vi "APSxSensorRefCurveLeveling.vi"(8 "error in (no error)":errorcluster caption="错误输入（无错误）", 9 "Param2":dbl, 10 "Param1":enum16{"APSX_PREV_INDEX_POINT_CALIBRATION"}(ring), 11 "hSENSOR":i32) -> (0 "error out":errorcluster caption="错误输出")   [LabVIEW 2018]
doc: "该模板用于创建子VI。"
uses:
  APSx.dll/APSx.dll
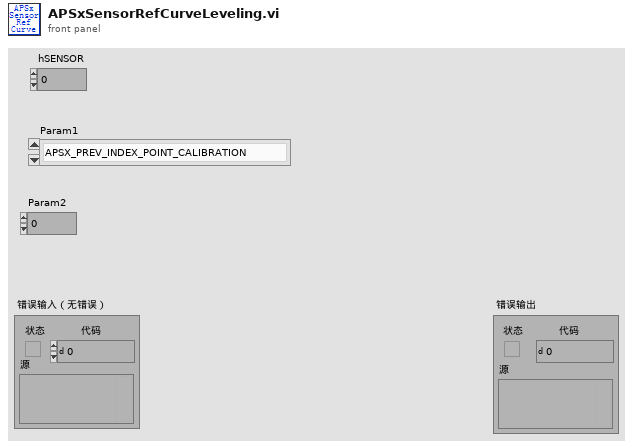
[diagram p1: front panel]
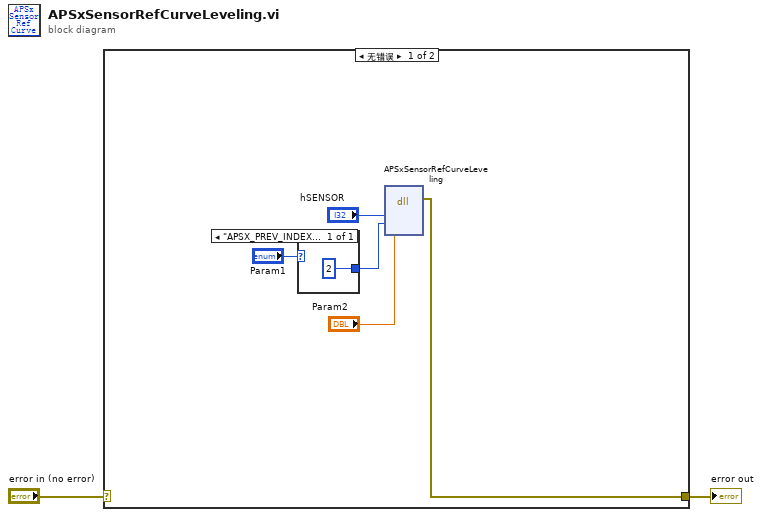
[diagram p0: block diagram]
diagram:
  n1 = case shown="无错误" "error in (no error)" {
    selector: "error in (no error)" -> [_ w9]
    tunnel: [w7 w9] -> w1
    frame No Error {
      n2 = case shown="\"APSX_PREV_INDEX_POINT_CALIBRATION\", 默认" "Param1" {
        tunnel: [2] -> w3
        frame "APSX_PREV_INDEX_POINT_CALIBRATION", Default {
        }
      }
      n3 = dll-call lib="PTH2]abs D项目Feng恒隆项目Labview传感器对中台SourcesAPSx.dllAPSx.dll" fn="APSxSensorRefCurveLeveling"("hSENSOR"="hSENSOR", "Param1"=w3, "Param2"="Param2") -> (error out=w7:errorcluster)  [unwired: 7 in, 1 out]
    }
    frame Error {
    }
  }
  "error out" <- w1
